vi "OpenTypedef-EditTime.vi"(6 "Mouse Position":T1, 7 "User VI Ref":refnum<vi>, 8 "Is Multi-select?":bool, 9 "Remaining Items":refnum<vi>[](array[refnum]), 10 "Affected Items":T8, 11 "Menu Refnum":refnum<k9>) -> (3 "Menu Items To Add":T2[](array[typedef]))   [LabVIEW 2020]
doc: "This VI is part of a plug-in for modifying the LabVIEW shortcut menus. This is the builder VI which is called when the shortcut menu is built. It tells LabVIEW which shortcut menu items to add to the menu."
uses:
  <resource>/plugins/PopupMenus/support/Checkmark Status.ctl
  <resource>/plugins/PopupMenus/support/Relative Position.ctl
  <resource>/plugins/PopupMenus/support/Position In Menu.ctl
  <resource>/plugins/PopupMenus/support/Transaction Control.ctl
  <resource>/plugins/PopupMenus/support/Shortcut Menu Item Definition.ctl
  <resource>/plugins/PopupMenus/support/Enabled Menu Item Status.ctl
  <vilib>/Utility/Data Type/Type Definitions/Data Type.ctl
  <vilib>/Utility/Data Type/NI_Data Type.lvlib
  b08720a3-ec3f-4dbd-bfcb-a13bd0ba3fe2.vi
  OpenTypedef-EditTime.ctl
  <vilib>/Utility/miscctls.llb/LVPositionTypeDef.ctl
panel:
  # "Rules a popup plug-in must follow:\n* This VI's file name must match the file name of the LLB -- only the file extensions should be different.\n* This VI must have debugging disabled or it will be ignored as a plug-in.\n* For all menu items, \"tag suffix + file name of this VI\" must be less than 240 characters.\n* You can disconnect the \"Affected Items\" from the typedef to make the plug-in load faster. The typedef is only there to assist you in keeping this VI and the execution VI using to the same type.\n* All controls on this panel except \"Affected Items\" are locked to prevent accidental edits. Do not change the types or the names of controls other than the elements inside the \"Affected Items\" cluster.\n* See Context Help for more information on the individual controls."
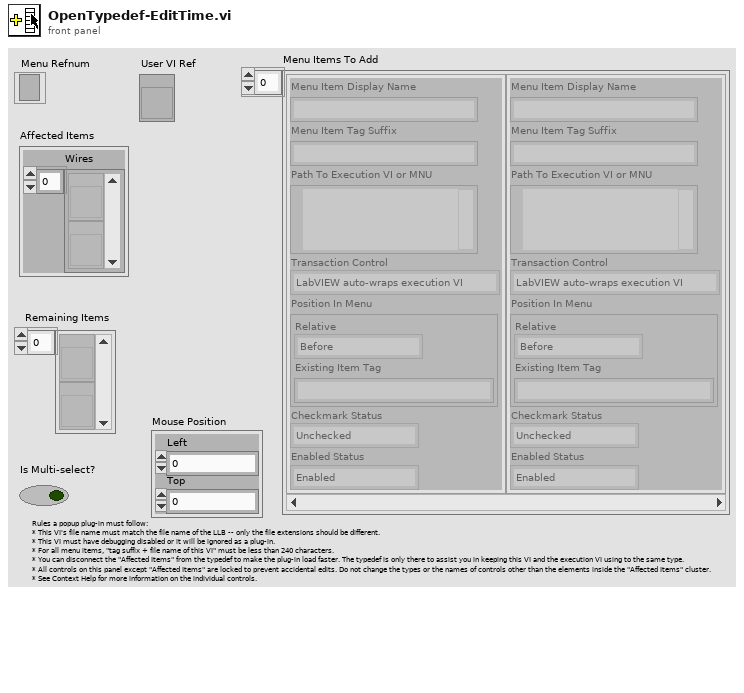
[diagram p1: front panel]
types:
  T1 = typedef "LVPositionTypeDef.ctl" = cluster{"Left":i32, "Top":i32}
  T2 = typedef "Shortcut Menu Item Definition.ctl" = cluster{"Menu Item Display Name":string, "Menu Item Tag Suffix":string, "Path To Execution VI or MNU":path, "Transaction Control":T3, "Position In Menu":T4, "Checkmark Status":T6, "Enabled Status":T7}
  T3 = typedef "Transaction Control.ctl" = enum8{"LabVIEW auto-wraps execution VI", "Execution VI will define if needed"}
  T4 = typedef "Position In Menu.ctl" = cluster{"Relative":T5, "Existing Item Tag":string}
  T5 = typedef "Relative Position.ctl" = enum8{"Before", "Instead of", "After", "Into Submenu"}
  T6 = typedef "Checkmark Status.ctl" = enum8{"Unchecked", "Checked"}
  T7 = typedef "Enabled Menu Item Status.ctl" = enum8{"Enabled", "Disabled"}
  T8 = typedef "OpenTypedef-EditTime.ctl" = cluster{"Wires":refnum<vi>[]}
  T9 = typedef "NI_Data Type.lvlib/Data Type.ctl" = enum8{"Invalid Type", "Void", "I8", "I16", "I32", "I64", "U8", "U16", "U32", "U64", "Single Float", "Double Float", "Extended Float", "Single Complex", "Double Complex", "Extended Complex", "Enum U8", "Enum U16", "Enum U32", "Enum U64", "Single Float With Unit", "Double Float With Unit", "Extended Float With Unit", "Single Complex with Unit", "Double Complex with Unit", "Extended Complex with Unit", "Boolean", "String", "Path", "Picture", "Tag", "Array", "Cluster", "Variant", "LV Variant", "Waveform", "Timestamp", "Digital Waveform", "Digital Data", "ExpressData", "Refnum", "External Data", "VI", "Poly VI", "LabVIEW Class Instance", "Fixed Point", "Set Collection", "Map Collection"}
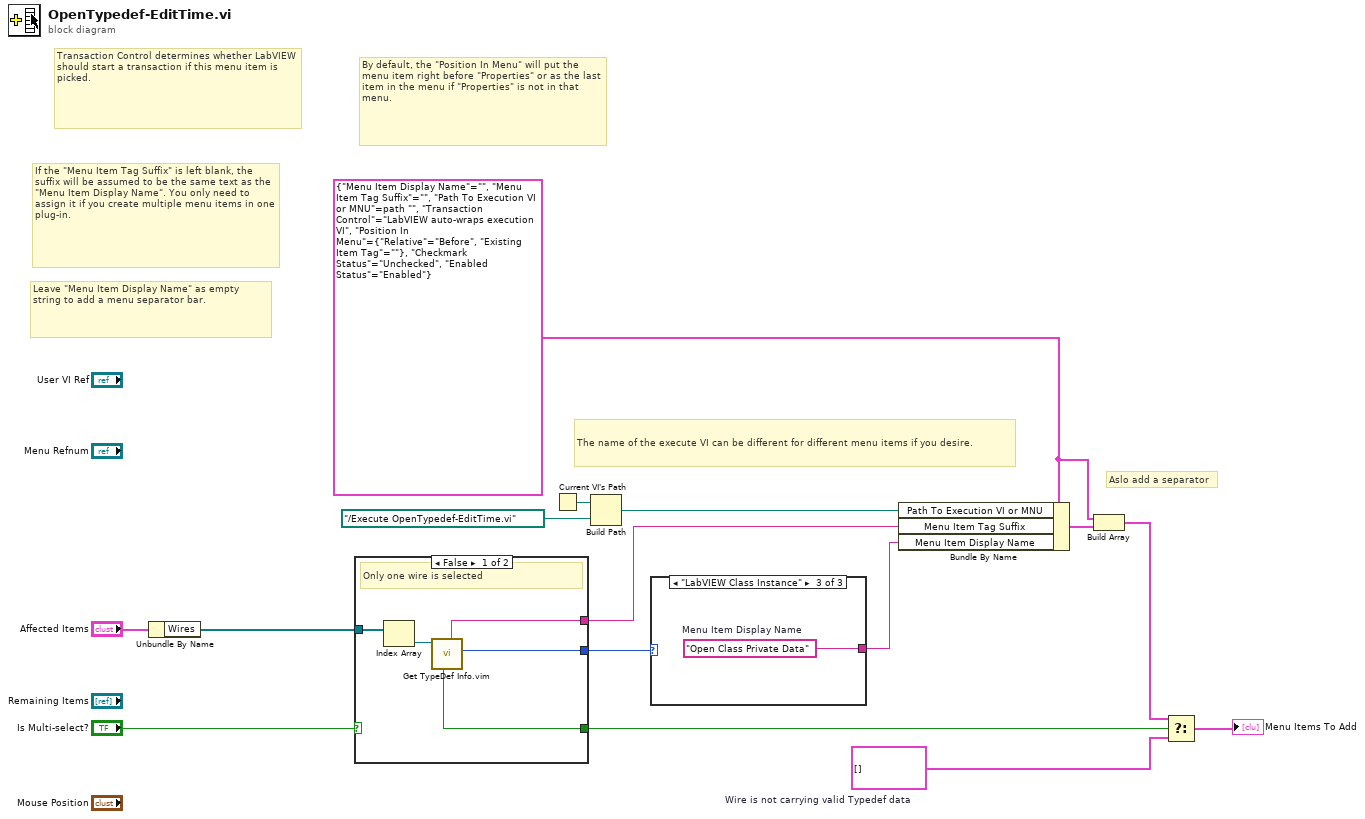
[diagram p0: block diagram]
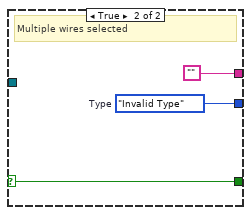
[diagram p2: hidden frame]
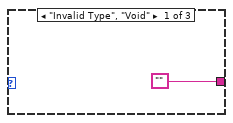
[diagram p3: hidden frame]
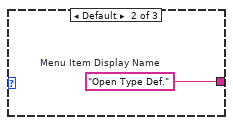
[diagram p4: hidden frame]
diagram:
  w6 = T2[] []  # Wire is not carrying valid Typedef data
  w2 = T2 {"Menu Item Display Name"="", "Menu Item Tag Suffix"="", "Path To Execution VI or MNU"=path "", "Transaction Control"=enum."LabVIEW auto-wraps execution VI", "Position In Menu"={"Relative"=enum."Before", "Existing Item Tag"=""}, "Checkmark Status"=enum."Unchecked", "Enabled Status"=enum."Enabled"} ("Cluster")
  # "Aslo add a separator"
  # "Transaction Control determines whether LabVIEW should start a transaction if this menu item is picked."
  # "Leave \"Menu Item Display Name\" as empty string to add a menu separator bar."
  # "If the \"Menu Item Tag Suffix\" is left blank, the suffix will be assumed to be the same text as the \"Menu Item Display Name\". You only need to assign it if you create multiple menu items in one plug-in."
  # "By default, the \"Position In Menu\" will put the menu item right before \"Properties\" or as the last item in the menu if \"Properties\" is not in that menu."
  # "The name of the execute VI can be different for different menu items if you desire."
  n1 = Unbundle By Name("Affected Items") -> ("Wires"=w10:refnum<vi>[])
  n2 = case shown="False" "Is Multi-select?" {
    selector: "Is Multi-select?" -> [_ w23]
    tunnel: w10 -> [w20 _]
    tunnel: [w16 w23] -> w9
    tunnel: [w17 ""] -> w5
    tunnel: [w18 w21] -> w3
    frame False {
      # "Only one wire is selected"
      n3 = Index Array(array=w20) -> (element=w19:refnum<vi>)  [unwired: 1 in]
      n4 = call "Get TypeDef Info.vim"("Ref in"=w19) -> ("Type"=w18:T9, "Type Definition/Class Path"=w17:string, "Typedef/Class Data?"=w16:bool)  [unwired: 4 in, 2 out]
    }
    frame True {
      w21 = Data_Type."Invalid Type"  # Type
      # "Multiple wires selected"
    }
  }
  n5 = Current VI's Path() -> (path=w12:path)
  n6 = Build Path(base path=w12, name or relative path=path "../Execute OpenTypedef-EditTime.vi" ("execute path")) -> (appended path=w14:path)
  n7 = case shown="\"LabVIEW Class Instance\"" w3 {
    tunnel: ["" w25 w26] -> w4
    frame "Invalid Type", "Void" {
    }
    frame Default {
      w25 = "Open Type Def."  # Menu Item Display Name
    }
    frame "LabVIEW Class Instance" {
      w26 = "Open Class Private Data"  # Menu Item Display Name
    }
  }
  n8 = Bundle By Name(cluster=w2, "Path To Execution VI or MNU"=w14, "Menu Item Tag Suffix"=w5, "Menu Item Display Name"=w4) -> (w13:T2)
  n9 = Build Array(w2, w13) -> (w8:T2[])
  n10 = Select(t=w8, s=w9, f=w6) -> (s? t:f=→"Menu Items To Add":T2[])
